vi "Write CCD Config.vi"(8 "error in (no error)":errorcluster, 10 "CCD Config":T1={"Exposure Time"=0.0, "Pre-amp gain"=0, "Readout Rate"=0, "EM Mode"=0, "EM Gain"=2, "Binning"=1, "Initial Line"=1, "Initial Cloumn"=1, "Final Line"=1024, "Final Column"=1024, "Kinetic Series Length"=0, "Shutter Mode"=2, "Cooler ON/OFF"=0, "Temperature"=20, "Image Name"="", "Image Path"="", "# Images"=1, "#index"=0} {"# Images" min=1; "Temperature" min=0 max=0; "Cooler ON/OFF" items=["Cooler OFF", "Cooler ON"]; "Shutter Mode" items=["Fully Auto", "OPEN", "CLOSED"]; "EM Mode" items=["Electron Multiplying", "Conventional"]; "Readout Rate" items=["1 MHz", "10 MHz", "20 MHz", "30 MHz"]; "Pre-amp gain" items=["Gain 1", "Gain 2"]}, 11 "Interface in":refnum<class "Interface.lvclass">) -> (0 "error out":errorcluster, 3 "Interface out":refnum<class "Interface.lvclass">)   [LabVIEW 2018, in "Interface.lvclass"]
uses:
  Interface.lvclass
  Interface.lvclass/Interface.ctl
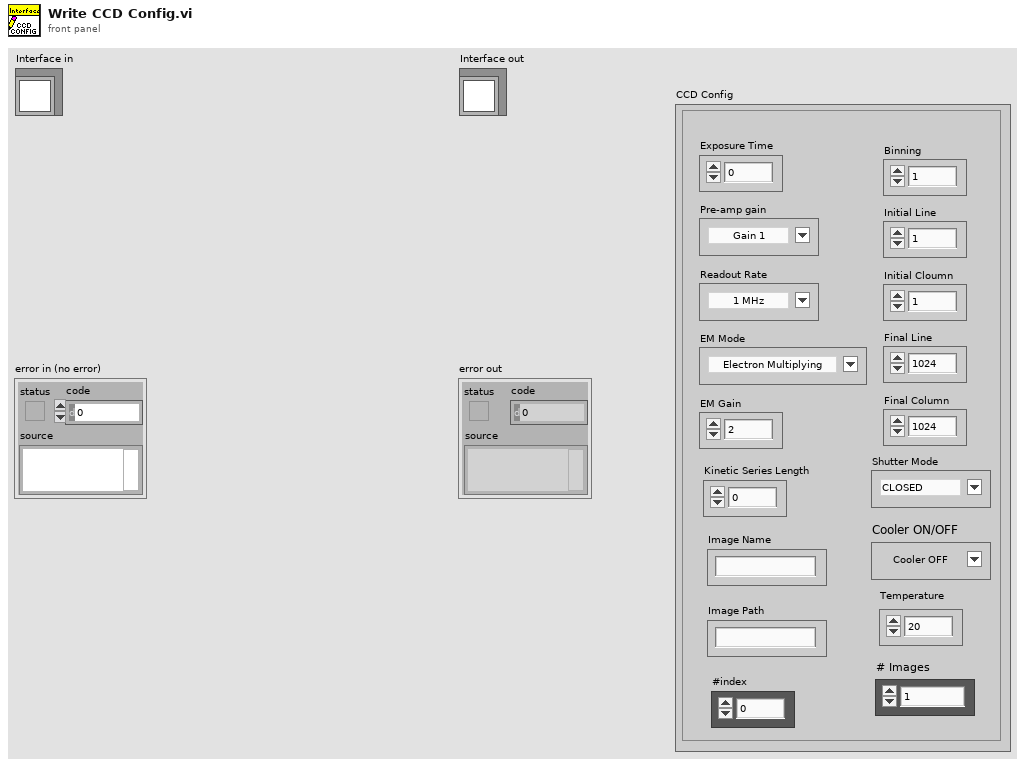
[diagram p1: front panel]
types:
  T1 = cluster{"Exposure Time":sgl, "Pre-amp gain":u8, "Readout Rate":u8, "EM Mode":u8, "EM Gain":u16, "Binning":u16, "Initial Line":u16, "Initial Cloumn":u16, "Final Line":u16, "Final Column":u16, "Kinetic Series Length":u32, "Shutter Mode":u8, "Cooler ON/OFF":u16, "Temperature":i8, "Image Name":string, "Image Path":string, "# Images":u32, "#index":u16}
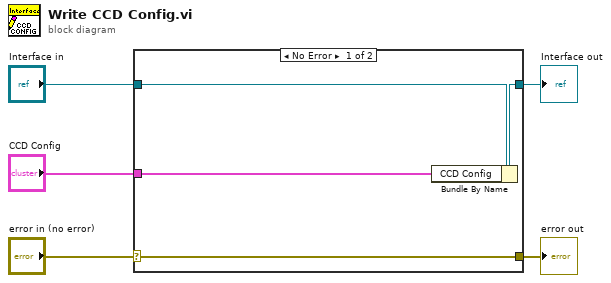
[diagram p0: block diagram]
diagram:
  n1 = case shown="No Error" "error in (no error)" {
    selector: "error in (no error)" -> [w9 w10]
    tunnel: [w9 w10] -> w4
    tunnel: [w7 w11] -> w2
    tunnel: "Interface in" -> [w8 w11]
    tunnel: "CCD Config" -> [w6 _]
    frame No Error {
      n2 = Bundle By Name(cluster=w8, "CCD Config"=w6) -> (w7:refnum<class "Interface.lvclass">)
    }
    frame Error {
    }
  }
  "error out" <- w4
  "Interface out" <- w2
